vi "Stop Core.vi"(10 "final error code":i32, 11 "Sample Line in":refnum<class "Sample Line.lvclass">) -> (3 "Sample Line out":refnum<class "Sample Line.lvclass">)   [LabVIEW 2015, in "cRIO-Carbondioxide.lvlib" / "CO2-Actor.lvlib" / "Sample Line.lvclass"]
doc: "(<B>Filename</B>: Actor Framework.lvlib:Actor.lvclass:Stop Core.vi)\n\nDefines what the actor does before it stops. Use the <B>final error code</B> input to determine whether the actor shut down in response to an error.\n\nBy default, this method does nothing. A descendant class may override it to define behavior, such as shutting down any processes the actor initiated in its override of the Actor Core method."
uses:
  Sample Line.lvclass
  Sample Line.lvclass/Sample Line.ctl
  <vilib>/ActorFramework/Message Enqueuer/Message Enqueuer.lvclass/Message Enqueuer.ctl
  <vilib>/ActorFramework/Message Enqueuer/Enqueue.vi
  <vilib>/ActorFramework/Message Priority Queue/Priority Enqueue.vi
  <vilib>/ActorFramework/Stop Msg/Stop Msg.lvclass
  CO2 Actor/CO2 Actor.lvclass
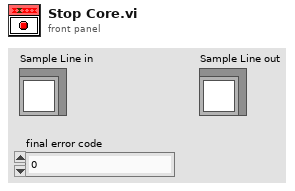
[diagram p1: front panel]
types:
  T1 = cluster{"Valve 1":refnum<class "Message Enqueuer.lvclass">, "Valve 2":refnum<class "Message Enqueuer.lvclass">, "Valve 3":refnum<class "Message Enqueuer.lvclass">, "Valve 4":refnum<class "Message Enqueuer.lvclass">, "Valve 5":refnum<class "Message Enqueuer.lvclass">}
  T2 = cluster{"Sample Line Control":refnum<k21>, "Sample Line Status":refnum<k21>}
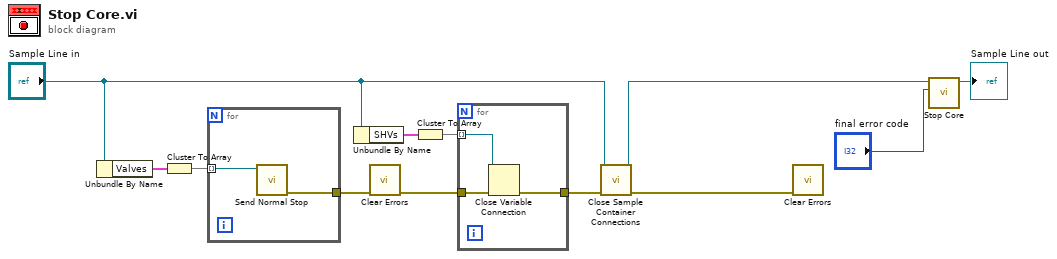
[diagram p0: block diagram]
diagram:
  n1 = Unbundle By Name("Sample Line in") -> ("Valves"=w8:T1)
  n2 = Cluster To Array(cluster=w8) -> (array=w9:refnum<class "Message Enqueuer.lvclass">[])
  n3 = for {
    tunnel: w9 -> [w14] mode=indexing
    tunnel: [w13] -> w10
    n4 = call <vilib>:"Send Normal Stop.vi"("Message Enqueuer"=w14) -> ("error out"=w13:errorcluster)  [unwired: 10 in]
  }
  n5 = Unbundle By Name("Sample Line in") -> ("SHVs"=w7:T2)
  n6 = call <vilib>:"Clear Errors.vi"("error in (no error)"=w10) -> ("error out"=w5:errorcluster)  [unwired: 5 in, 1 out]
  n7 = Cluster To Array(cluster=w7) -> (array=w6:refnum<k21>[])
  n8 = for {
    tunnel: w6 -> [w17] mode=indexing
    tunnel: [w16] -> w3
    tunnel: w5 -> [w15]
    n9 = Close Variable Connection(8:w15, 11:w17) -> (0:w16:errorcluster)
  }
  n10 = call "Close Sample Container Connections.vi"("error in (no error)"=w3, "Sample Line in"="Sample Line in") -> ("error out"=w1:errorcluster, "Sample Line out"=w2:refnum<class "Sample Line.lvclass">)  [unwired: 8 in]
  n11 = call <vilib>:"Clear Errors.vi"("error in (no error)"=w1) -> ()  [unwired: 5 in, 2 out]
  n12 = call-parent "Stop Core.vi"("final error code"="final error code", "CO2 Actor in"=w2) -> ("CO2 Actor out"=→"Sample Line out":refnum<class "Sample Line.lvclass">)  [unwired: 9 in]
